vi "User_Defined_Test_Hash String to Numeric.vi"(8 "error in (no error)":errorcluster) -> (0 "error out":errorcluster, 3 "Unit Test Framework Results":T1)   [LabVIEW 2023]
doc: "Use this template to create a user-defined test VI. Define your test requirements and wire the results to the <b>Result (Test)</b> control. Do not modify the <b>Unit Test Framework Results</b> indicator."
uses:
  <vilib>/utf/common/utf_test_comparison_operators.ctl
  <vilib>/utf/NI_UnitTestFramework.lvlib
  <vilib>/utf/common/utf_test_result.ctl
  <vilib>/utf/common/utf_test_result_failure.ctl
  <vilib>/utf/common/utf_test_result_troll.ctl
  <vilib>/utf/common/utf_vi_tag.ctl
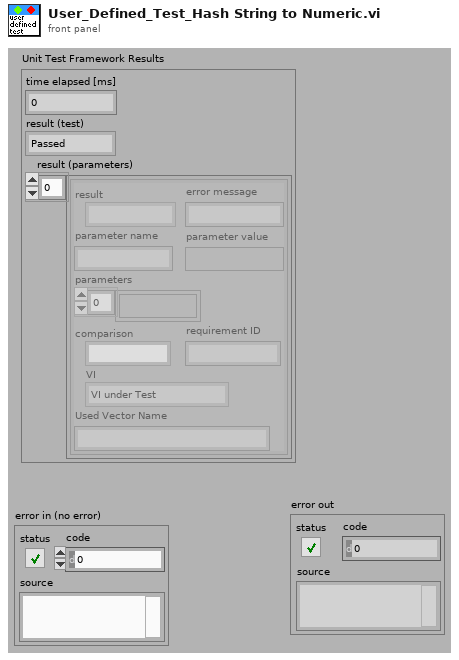
[diagram p1: front panel]
types:
  T1 = typedef "NI_UnitTestFramework.lvlib/utf_test_result_troll.ctl" = cluster{"time elapsed [ms]":u32, "result (test)":T2, "result (parameters)":T3[]}
  T2 = typedef "NI_UnitTestFramework.lvlib/utf_test_result.ctl" = enum16{"Passed", "Failed", "Error", "Skipped", "Not Processed"}
  T3 = typedef "NI_UnitTestFramework.lvlib/utf_test_result_failure.ctl" = cluster{"result":T2, "error message":string, "parameter name":string, "parameter value":variant, "parameters":variant[], "comparison":T4, "requirement ID":string, "VI":T5, "Used Vector Name":string}
  T4 = typedef "NI_UnitTestFramework.lvlib/utf_test_comparison_operators.ctl" = enum16{"=", "!=", ">", ">=", "<", "<=", "range", "symmetric tolerance", "asymmetric tolerance", "string contains", "string not contain", "array size", "string length", "array range", "by element", "array range (limit array)", "user-defined", "array contains", "array not contain", "vector length", "= (elm)", "!= (elm)", "= (case insensitive)", "!= (case insensitive)"}
  T5 = typedef "NI_UnitTestFramework.lvlib/utf_vi_tag.ctl" = enum16{"Setup VI", "VI under Test", "Teardown VI"}
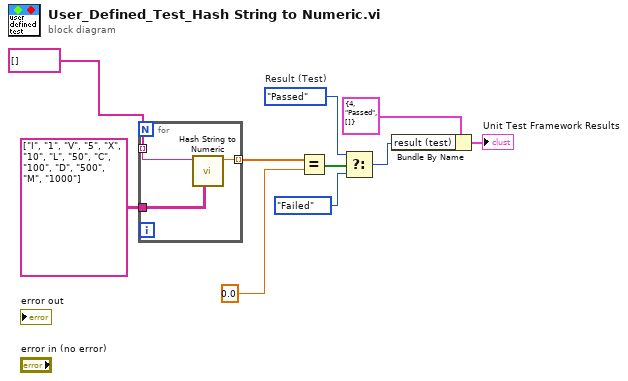
[diagram p0: block diagram]
diagram:
  w7 = utf_test_result."Passed"  # Result (Test)
  n1 = for {
    tunnel: string[][] [["I", "1"], ["V", "5"], ["X", "10"], ["L", "50"], ["C", "100"], ["D", "500"], ["M", "1000"]] -> [w13]
    tunnel: [w12] -> w3 mode=indexing
    tunnel: string[] [] -> [w11] mode=indexing
    n2 = call "Hash String to Numeric.vi"("Hash Array"=w13, "String Input"=w11) -> ("Numeric Output"=w12:dbl)  [unwired: 8 in, 1 out]
  }
  n3 = Equal?(x=w3, y=0.0) -> (x = y?=w4:bool[])
  n4 = Select(t=w7, s=w4, f=utf_test_result."Failed") -> (s? t:f=w5:T2)
  n5 = Bundle By Name(cluster=T1 {"time elapsed [ms]"=4, "result (test)"=enum."Passed", "result (parameters)"=[]} ("Unit Test Framework - Result"), "result (test)"=w5) -> (→"Unit Test Framework Results":T1)
